vi "Turn Angle to Drive Distance.vi"(5 "Wheelbase (in)":dbl=21.5, 9 "Angle (rads)":dbl) -> (3 "Distance (in)":dbl)   [LabVIEW 2015]
panel:
  # "Arc Length = r * Theta\nr = 1/2 * wheel base"
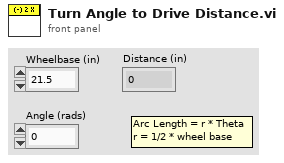
[diagram p1: front panel]
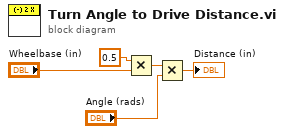
[diagram p0: block diagram]
diagram:
  n1 = Multiply(x=0.5, y="Wheelbase (in)") -> (x*y=w2:dbl)
  n2 = Multiply(x=w2, y="Angle (rads)") -> (x*y=→"Distance (in)":dbl)
